vi "2pi_grises.vi"(8 "error in (no error)":errorcluster, 10 "Puerto":refnum<visa-resource-name>="COM2", 11 "Cam Session":T1 caption="Session Out") -> (0 "error out":errorcluster, 3 "V 2Pi\nActual":sgl=3.4309938 format="%#.1g")   [LabVIEW 2020]
uses:
  <vilib>/userdefined/High Color/IMAQdx.ctl
  Controls/Calib states --- typedef.ctl
  Controls/Calib data ---typedef.ctl
  <vilib>/vision/Image Controls.llb/IMAQ Image.ctl
  64c00cdc-7401-4ced-a99b-d285ba44592a.vi
  <vilib>/Instr/_visa.llb/VISA Configure Serial Port (Instr).vi
  <vilib>/vision/driver/NI_Vision_Acquisition_Software.lvlib
  <vilib>/vision/NI_Vision_Development_Module.lvlib
panel:
  out "Last Mouse Position:All Elements":cluster{"X":i32, "Y":i32}
  in  "Sust":bool=TRUE caption="Sustraer?"
  in  "dV (V)":sgl=0.4 min=0.1 max=5 step=0.1 format="%.1f"
  in  "dt (ms)":u32=5
  in  "Rango (V)":u8=7 max=100 step=1
  in  "Canal":string="X"
  in  "Cancelar":bool
  in  "V 2Pi\nApriori":sgl=4.0 min=0.1 max=15 step=0.1 format="%.1f"
  in  "Selección Rectángulo (px)":T2={"Left"=80, "Top"=180, "Right"=730, "Bottom"=830}
  out "valor enviado":string="17.2"
  in  "Iniciar":bool
  out "Captura":T3(plugin-control)
  out "tiempo total":u32=1016
  out "Ciclos 2Pi":cluster{"xi used":dbl[], "yi":dbl[]}[](graph)=[{"xi used"=[0.0, 0.4000000059604645, 0.800000011920929, 1.2000000476837158, 1.600000023841858, 2.0, 2.4000000953674316, 2.799999952316284, 3.200000047683716, 3.6000001430511475, 4.0, 4.400000095367432, 4.800000190734863, 5.200000286102295, 5.599999904632568, 6.0, 6.400000095367432, 6.800000190734863, 7.200000286102295], "yi"=[1.6194082498550415, 2.081223726272583, 3.9639101028442383, 5.417988300323486, 5.994996547698975, 5.763517379760742, 4.927460193634033, 3.268064022064209, 1.9228070974349976, 2.006049633026123, 3.322584629058838, 5.178757190704346, 5.874281883239746, 5.9817633628845215, 5.3586106300354, 3.7743194103240967, 2.4187028408050537, 2.3153183460235596, 3.7917206287384033]}, {"xi used"=[0.0, 0.10000000149011612, 0.20000000298023224, 0.30000000447034836, 0.4000000059604645, 0.5000000074505806, 0.6000000089406967, 0.7000000104308128, 0.800000011920929, 0.9000000208616257, 1.0000000298023224, 1.100000038743019, 1.2000000476837158, 1.3000000417232513, 1.4000000357627869, 1.5000000298023224, 1.600000023841858, 1.7000000178813934, 1.800000011920929, 1.9000000059604645, 2.0, 2.100000023841858, 2.200000047683716, 2.3000000715255737, 2.4000000953674316, 2.5000000596046448, 2.600000023841858, 2.699999988079071, 2.799999952316284, 2.899999976158142, 3.0, 3.100000023841858, 3.200000047683716, 3.3000000715255737, 3.4000000953674316, 3.5000001192092896, 3.6000001430511475, 3.7000001072883606, 3.8000000715255737, 3.900000035762787, 4.0, 4.100000023841858, 4.200000047683716, 4.300000071525574, 4.400000095367432, 4.5000001192092896, 4.6000001430511475, 4.700000166893005, 4.800000190734863, 4.900000214576721, 5.000000238418579, 5.100000262260437, 5.200000286102295, 5.300000190734863, 5.400000095367432, 5.5, 5.599999904632568, 5.699999928474426, 5.799999952316284, 5.899999976158142, 6.0, 6.100000023841858, 6.200000047683716, 6.300000071525574, 6.400000095367432, 6.5000001192092896, 6.6000001430511475, 6.700000166893005, 6.800000190734863, 6.900000214576721, 7.000000238418579, 7.100000262260437, 7.200000286102295], "yi"=[1.6194082498550415, 1.6415202646400873, 1.700969021152869, 1.835091261121122, 2.081223726272583, 2.4615675244221595, 2.9377812277334487, 3.4563877744572187, 3.9639101028442383, 4.416314498578613, 4.807340439884618, 5.1401707620402455, 5.417988300323486, 5.643229129866736, 5.815342479071086, 5.9330308007455095, 5.994996547698975, 6.0015645873541725, 5.959549445588673, 5.8773880628937665, 5.763517379760742, 5.622745854472534, 5.4453682711596425, 5.218050945615625, 4.927460193634033, 4.566549653810085, 4.153420905030226, 3.7124627576598135, 3.268064022064209, 2.8442846434260165, 2.4638706226251452, 2.1492390703865025, 1.9228070974349976, 1.8016579460584699, 1.7815393847964844, 1.8528653137515367, 2.006049633026123, 2.2327082258196134, 2.529265762805696, 2.8933489839101707, 3.322584629058838, 3.807336769827714, 4.308917005977046, 4.78137419407865, 5.178757190704346, 5.467236063197128, 5.661465721984701, 5.788222288265946, 5.874281883239746, 5.940712665430707, 5.985750942666336, 6.001925060099863, 5.9817633628845215, 5.9173299887642, 5.798831744986865, 5.616011126946077, 5.3586106300354, 5.0225638976458455, 4.628571701943094, 4.203526165358669, 3.7743194103240967, 3.3657338746848104, 2.994113257941885, 2.673691575010305, 2.4187028408050537, 2.2430304554985607, 2.1591553602930404, 2.1792078816481535, 2.3153183460235596, 2.5722541809073114, 2.925331217901028, 3.3425023896347215, 3.7917206287384033]}, {"xi used"=[1.6635191881348852, 5.094512955533968], "yi"=[6.004797437208987, 6.001979760925586]}]
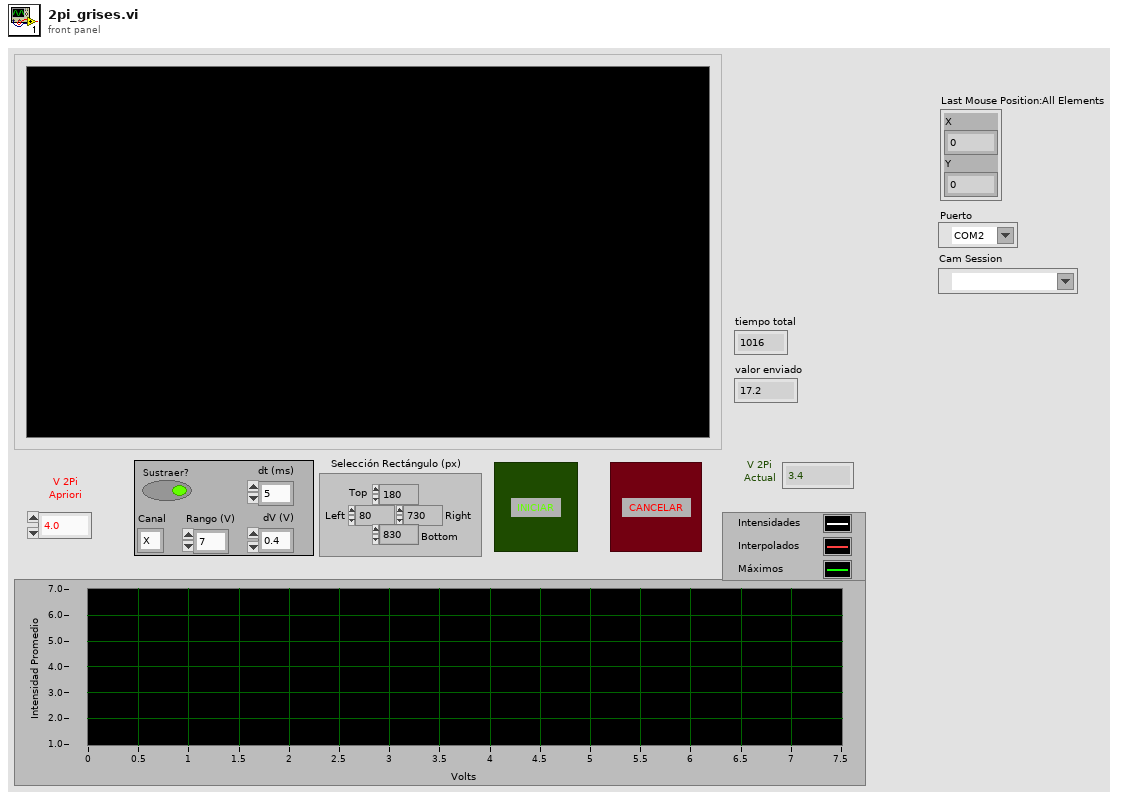
[diagram p1: front panel]
types:
  T1 = typedef "IMAQdx.ctl" = refnum<k21>
  T2 = cluster{"Left":i32, "Top":i32, "Right":i32, "Bottom":i32}
  T3 = typedef "IMAQ Image.ctl" = refnum<image>
  T4 = typedef "Calib data ---typedef.ctl" = cluster{"t0":u32, "Voltage":sgl[], "Mean pix value":sgl[], "Rectangle":cluster{"Left":i32, "Top":i32, "Right":i32, "Bottom":i32}, "New calibration?":bool, "Images":T3[]}
  T5 = typedef "Calib states --- typedef.ctl" = enum16{"Init", "Wait", "Aqcuire base image", "Aquire and process", "Calculate results", "Prompt to repeat", "Clear buffers", "Exit"}
  T6 = typedef "lveventtype.ctl" = enum32{"Null", "Timeout", "Annotation Menu Selection", "Annotation Menu Selection?", "App Instance Close", "App Instance Close?", "Autoscale Range Change", "Bookmark Info Change", "Cell Edit", "Cell Edit?", "Cursor Grab", "Cursor Grab?", "Cursor Menu Selection", "Cursor Menu Selection?", "Cursor Move", "Cursor Release", "Data Change", "Direction Change", "Display State Change", "Drag Ended", "Drag Enter", "Drag Leave", "Drag Over", "Drag Source Update", "Drag Starting", "Drag Starting?", "Drop", "Exec State Change", "Key Down", "Key Down?", "Key Repeat", "Key Repeat?", "Key Up", "Listbox Double Click", "Menu Activation?", "Menu Selection (App)", "Menu Selection? (App)", "Menu Selection (User)", "Mouse Down", "Mouse Down?", "Mouse Enter", "Mouse Leave", "Mouse Move", "Mouse Up", "Mouse Wheel", "NI Security User Change (App)", "Pane Size", "Panel Close", "Panel Close?", "Panel Resize", "Plot Attribute Change", "Scale Range Change", "Shortcut Menu Activation?", "Shortcut Menu Selection (App)", "Shortcut Menu Selection? (App)", "Shortcut Menu Selection (User)", "Tree Double Click", "Tree Drag", "Tree Drag?", "Tree Drop", "Tree Drop?", "Tree Item Close", "Tree Item Close?", "Tree Item Open", "Tree Item Open?", "User Event", "Value Change"}
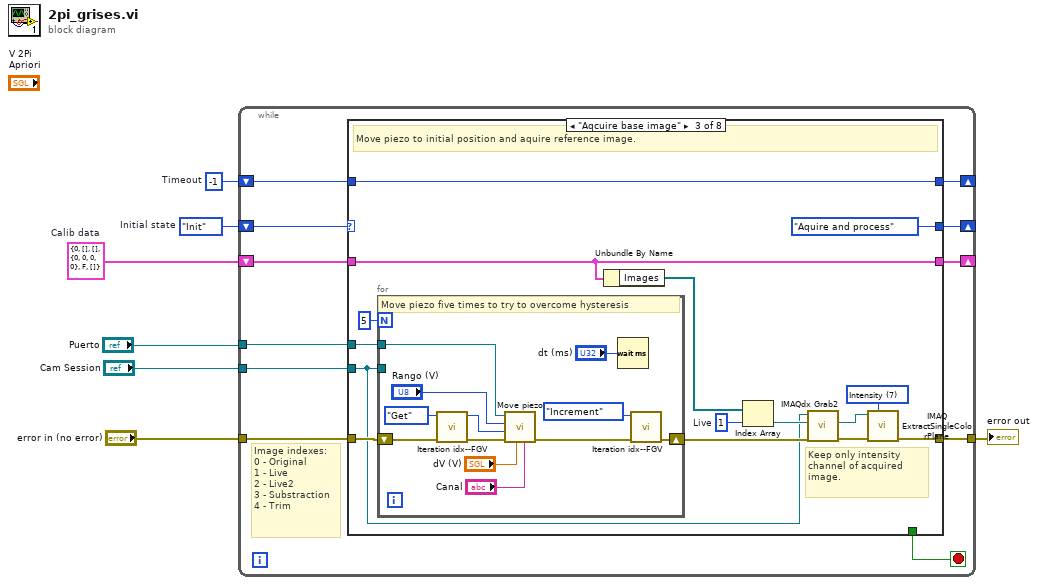
[diagram p0: block diagram]
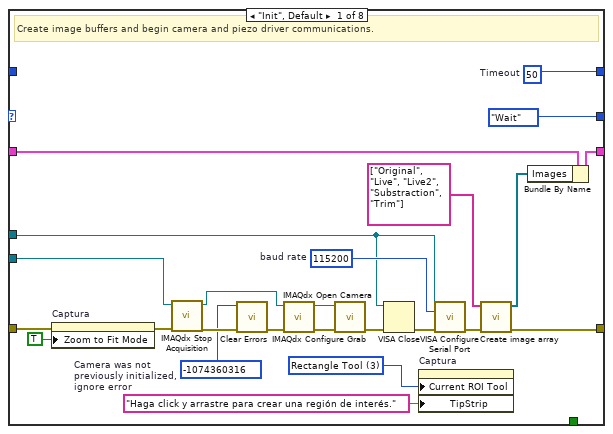
[diagram p2: hidden frame]
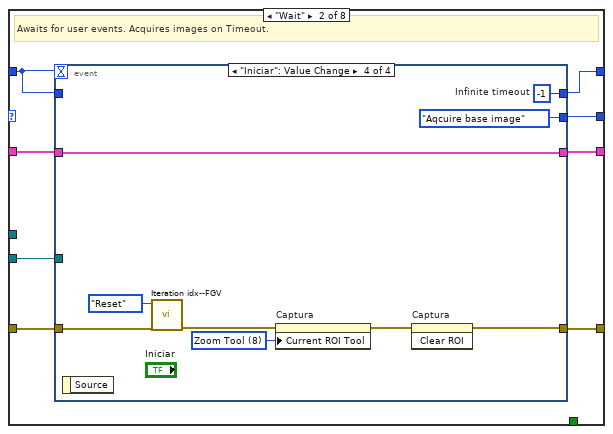
[diagram p3: hidden frame]
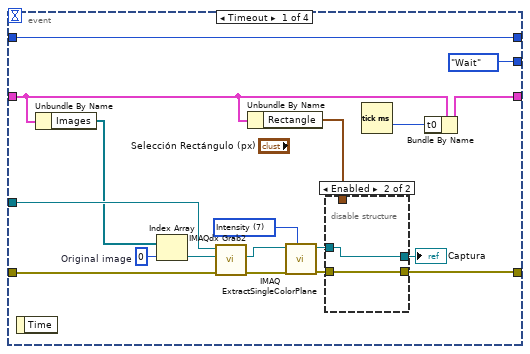
[diagram p4: hidden frame]
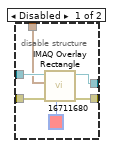
[diagram p5: hidden frame]
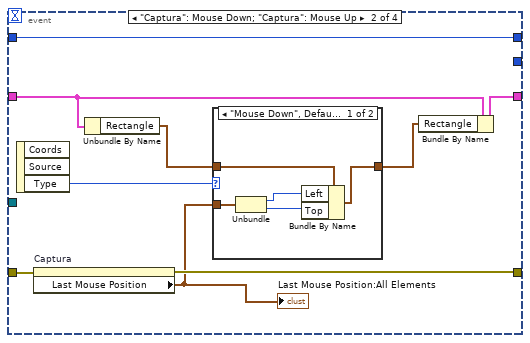
[diagram p6: hidden frame]
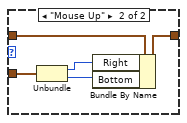
[diagram p7: hidden frame]
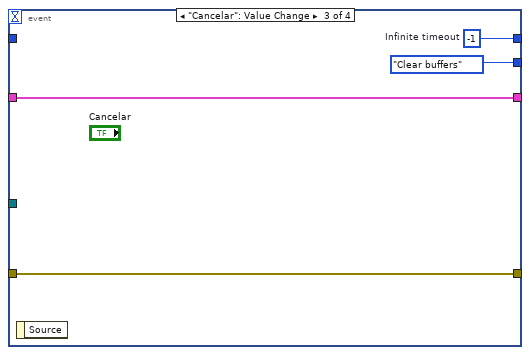
[diagram p8: hidden frame]
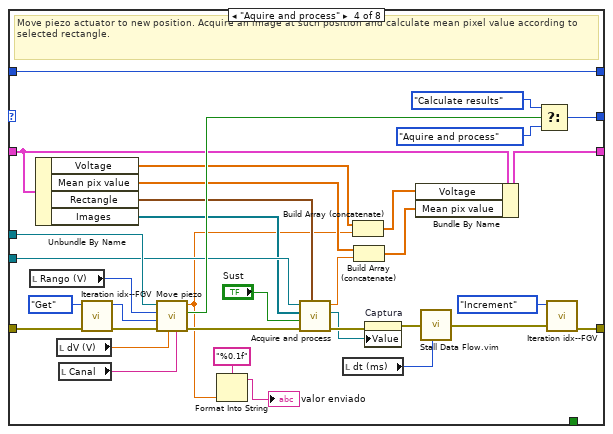
[diagram p9: hidden frame]
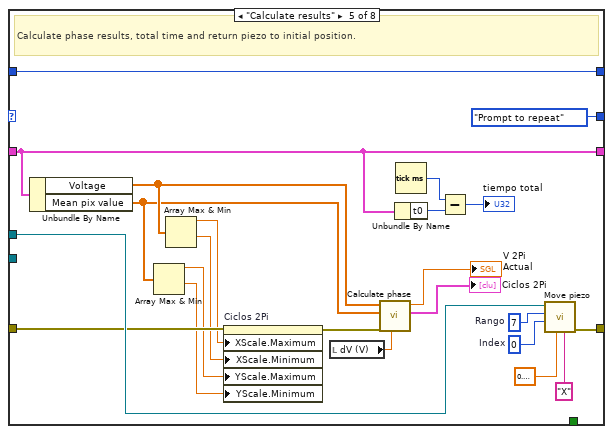
[diagram p10: hidden frame]
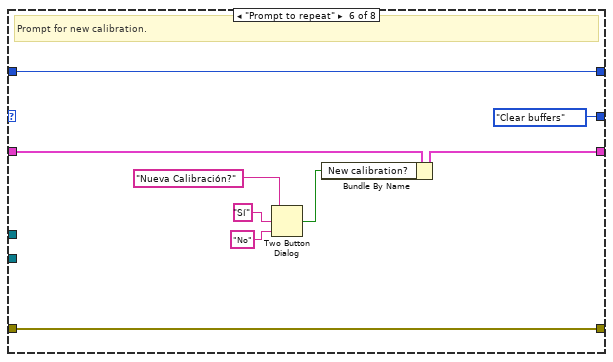
[diagram p11: hidden frame]
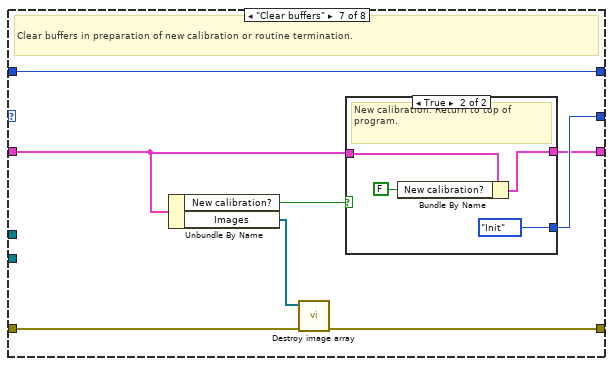
[diagram p12: hidden frame]
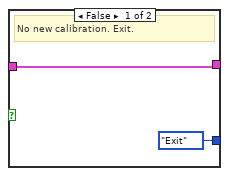
[diagram p13: hidden frame]
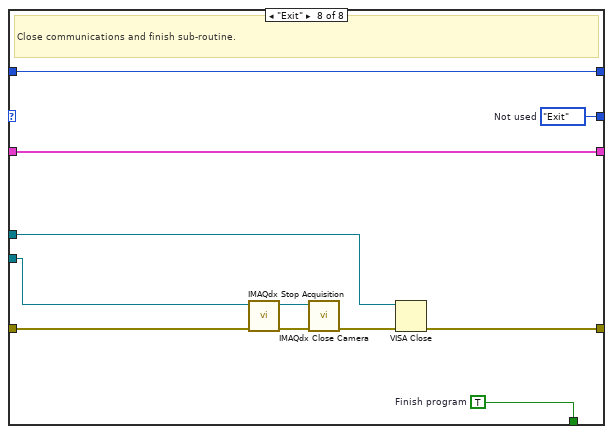
[diagram p14: hidden frame]
diagram:
  w2 = T4 {"t0"=0, "Voltage"=[], "Mean pix value"=[], "Rectangle"={"Left"=0, "Top"=0, "Right"=0, "Bottom"=0}, "New calibration?"=FALSE, "Images"=[]}  # Calib data
  w3 = -1  # Timeout
  w7 = Calib_states_---_typedef."Init"  # Initial state
  n1 = while {
    tunnel: [w16] -> w5
    tunnel: "error in (no error)" -> [w15]
    shift-right: [w14] -> _
    shift-left: w7 -> [w18]
    tunnel: "Cam Session" -> [w13]
    shift-right: [w11] -> _
    shift-left: w3 -> [w12]
    shift-right: [w10] -> _
    shift-left: w2 -> [w9]
    tunnel: "Puerto" -> [w8]
    stop <- w17 stop-if-true
    # "Image indexes:\n0 - Original\n1 - Live\n2 - Live2\n3 - Substraction\n4 - Trim"
    n2 = case shown="\"Aqcuire base image\"" w18 {
      tunnel: [_ _ _ _ _ _ _ w227] -> w17
      tunnel: [w26 w46 w112 w162 w184 w202 w208 w218] -> w16
      tunnel: w15 -> [w32 w47 w122 w168 w178 w202 w209 w223]
      tunnel: [Calib_states_---_typedef."Wait" w50 Calib_states_---_typedef."Aquire and process" ("Not used") w163 Calib_states_---_typedef."Prompt to repeat" ("Not used") Calib_states_---_typedef."Clear buffers" ("f") w210 w226] -> w14
      tunnel: w13 -> [w36 w45 w109 w157 _ _ _ w222]
      tunnel: w12 -> [_ w49 w123 w170 w193 w201 w207 w225]
      tunnel: [w33 w48 w123 w170 w193 w201 w207 w225] -> w11
      tunnel: [w22 w44 w111 w155 w188 w194 w204 w224] -> w10
      tunnel: w9 -> [w23 w43 w111 w154 w188 w196 w205 w224]
      tunnel: w8 -> [w24 _ w119 w169 w183 _ _ w217]
      frame "Init", Default {
        w20 = u32 3 items=["Zoom Tool"=8, "Selection Tool"=0, "Pan Tool"=9, "Point Tool"=1, "Line Tool"=2, "Rectangle Tool"=3, "Rotated Rectangle Tool"=12, "Polyline Tool"=10, "Polygon Tool"=5, "Freehand Tool"=11, "Closed Freehand Tool"=6, "Ellipse Tool"=4, "Annulus Tool"=7] ("Current ROI Tool")
        w30 = u32 115200  # baud rate
        w33 = 50  # Timeout
        w37 = -1074360316  # Camera was not previously initialized, ignore error
        # "Create image buffers and begin camera and piezo driver communications."
        n3 = property on="Captura" class="ImageControl"(error in=w32, "Zoom to Fit Mode"=TRUE) -> (error out=w28:errorcluster)  [unwired: 1 in, 1 out]
        n4 = call <vilib>:"IMAQdx Stop Acquisition.vi"("error in"=w28, "Session In"=w36) -> ("error out"=w40:errorcluster, "Session Out"=w38:T1)  [unwired: 8 in]
        n5 = call <vilib>:"Clear Errors.vi"("error in (no error)"=w40, "specific error code to clear (0: all)"=w37) -> ("error out"=w39:errorcluster)  [unwired: 4 in, 1 out]
        n6 = call <vilib>:"IMAQdx Open Camera.vi"("error in"=w39, "Session In"=w38) -> ("error out"=w35:errorcluster, "Session Out"=w34:T1)  [unwired: 8 in]
        n7 = call <vilib>:"IMAQdx Configure Grab.vi"("error in"=w35, "Session In"=w34) -> ("error out"=w29:errorcluster)  [unwired: 8 in, 1 out]
        n8 = VISA Close(VISA resource name=w24, error in (no error)=w29) -> (error out=w25:errorcluster)
        n9 = property on="Captura" class="ImageControl"("Current ROI Tool"=w20, "TipStrip"="Haga click y arrastre para crear una región de interés." ("Tip Strip")) -> ()  [unwired: 2 in, 2 out]
        n10 = call-poly "VISA Configure Serial Port"("VISA resource name"=w24, "baud rate (9600)"=w30, "error in (no error)"=w25) -> ("error out"=w27:errorcluster)  [unwired: 11 in, 1 out]
        n11 = call "Create image array.vi"("error in (no error)"=w27, "Name idx"=string[] ["Original", "Live", "Live2", "Substraction", "Trim"]) -> ("error out"=w26:errorcluster, "Image array"=w21:T3[])  [unwired: 8 in]
        n12 = Bundle By Name(cluster=w23, "Images"=w21) -> (w22:T4)
      }
      frame "Wait" {
        # "Awaits for user events. Acquires images on Timeout."
        n13 = event shown="[3] \"Iniciar\": Value Change" {
          selector: _ -> [_ _ _ _]
          dyn-events: _ -> [_ _ _ _]
          timeout: w49 -> [_ _ _ _]
          tunnel: [Calib_states_---_typedef."Wait" _ Calib_states_---_typedef."Clear buffers" Calib_states_---_typedef."Aqcuire base image"] -> w50
          tunnel: w49 -> [w67 w85 _ _]
          tunnel: [w67 w85 w96 w106] -> w48
          tunnel: w47 -> [w64 w84 w98 w104]
          tunnel: [w59 w83 w98 w100] -> w46
          tunnel: w45 -> [w63 _ _ _]
          tunnel: [w55 w78 w97 w108] -> w44
          tunnel: w43 -> [w52 w79 w97 w108]
          event Timeout {
            w53 = 7 items=["Red", "Green", "Blue", "Hue", "Saturation", "Luminance", "Value", "Intensity"] ("Color Plane")
            w66 = 0  # Original image
            n14 = event-data() -> ()  [unwired: 1 in, 1 out]
            n15 = Unbundle By Name(w52) -> ("Images"=w54:T3[])
            n16 = Index Array(array=w54, index=w66) -> (element=w65:T3)
            n17 = call <vilib>:"IMAQdx Grab2.vi"("error in"=w64, "Image In"=w65, "Session In"=w63) -> ("error out"=w60:errorcluster, "Image Out"=w57:T3)  [unwired: 5 in, 2 out]
            n18 = Unbundle By Name(w52) -> ("Rectangle"=w51:T2)
            n19 = call "IMAQ ExtractSingleColorPlane"("Color Plane"=w53, "error in (no error)"=w60, "Image Src"=w57) -> ("error out"=w62:errorcluster, "Image Dst Out"=w61:T3)  [unwired: 7 in]
            n20 = disable-structure shown="Enabled" {
              disable-tunnel: w62 -> [w74 w75]
              disable-tunnel: w61 -> [w73 w76]
              disable-tunnel: [w72 w75] -> w59
              disable-tunnel: [w71 w76] -> w58
              disable-tunnel: w51 -> [w69 _]
              frame Disabled {
                n21 = call "IMAQ Overlay Rectangle"("Color"=u32 16711680, "error in (no error)"=w74, "Rectangle"=w69, "Image"=w73) -> ("error out"=w72:errorcluster, "Image Out"=w71:T3)  [unwired: 6 in]
              }
              frame Enabled {
              }
            }
            "Captura" <- w58
            n22 = Tick Count (ms)() -> (millisecond timer value=w56:u32)
            n23 = Bundle By Name(cluster=w52, "t0"=w56) -> (w55:T4)
          }
          event "Captura": Mouse Down; "Captura": Mouse Up {
            n24 = event-data() -> ("Type"=w82:T6)  [unwired: 1 in, 2 out]
            n25 = property on="Captura" class="ImageControl"(error in=w84) -> (error out=w83:errorcluster, "Last Mouse Position"=w80:cluster{"X":i32, "Y":i32})  [unwired: 1 in, 1 out]
            "Last Mouse Position:All Elements" <- w80
            n26 = Unbundle By Name(w79) -> ("Rectangle"=w81:T2)
            n27 = case shown="\"Mouse Down\", Default" w82 {
              tunnel: w81 -> [w87 w94]
              tunnel: w80 -> [w88 w95]
              tunnel: [w86 w91] -> w77
              frame "Mouse Down", Default {
                n28 = Unbundle(w88) -> ("X"=w90:i32, "Y"=w89:i32)
                n29 = Bundle By Name(cluster=w87, "Left"=w90, "Top"=w89) -> (w86:T2)
              }
              frame "Mouse Up" {
                n30 = Unbundle(w95) -> ("X"=w93:i32, "Y"=w92:i32)
                n31 = Bundle By Name(cluster=w94, "Right"=w93, "Bottom"=w92) -> (w91:T2)
              }
            }
            n32 = Bundle By Name(cluster=w79, "Rectangle"=w77) -> (w78:T4)
          }
          event "Cancelar": Value Change {
            w96 = -1  # Infinite timeout
            n33 = event-data() -> ()  [unwired: 1 in, 1 out]
          }
          event "Iniciar": Value Change {
            w102 = u32 8 items=["Zoom Tool"=8, "Selection Tool"=0, "Pan Tool"=9, "Point Tool"=1, "Line Tool"=2, "Rectangle Tool"=3, "Rotated Rectangle Tool"=12, "Polyline Tool"=10, "Polygon Tool"=5, "Freehand Tool"=11, "Closed Freehand Tool"=6, "Ellipse Tool"=4, "Annulus Tool"=7] ("Current ROI Tool")
            w106 = -1  # Infinite timeout
            n34 = event-data() -> ()  [unwired: 1 in, 1 out]
            n35 = call "Iteration idx--FGV.vi"("error in (no error)"=w104, "Action"=enum16{"Reset", "Get", "Increment"}."Reset") -> ("error out"=w103:errorcluster)  [unwired: 8 in, 1 out]
            n36 = property on="Captura" class="ImageControl"(error in=w103, "Current ROI Tool"=w102) -> (error out=w101:errorcluster)  [unwired: 1 in, 1 out]
            n37 = invoke on="Captura" class="ImageControl" method="Clear ROI"(error in=w101) -> (error out=w100:errorcluster)  [unwired: 2 in, 2 out]
          }
        }
      }
      frame "Aqcuire base image" {
        w116 = 7 items=["Red", "Green", "Blue", "Hue", "Saturation", "Luminance", "Value", "Intensity"] ("Color Plane")
        w115 = 1  # Live
        # "Keep only intensity channel of acquired image."
        # "Move piezo to initial position and aquire reference image."
        n38 = for {
          N: 5 -> [_]
          tunnel: w109 -> [_]
          shift-right: [w133] -> w114
          shift-left: w122 -> [w132]
          tunnel: w119 -> [w128]
          # "Move piezo five times to try to overcome hysteresis"
          n39 = call "Iteration idx--FGV.vi"("error in (no error)"=w132, "Action"=enum16{"Reset", "Get", "Increment"}."Get") -> ("error out"=w130:errorcluster, "Index"=w124:i32)  [unwired: 8 in]
          n40 = call "Move piezo.vi"("Canal"="Canal", "dV"="dV (V)", "error in (no error)"=w130, "Index"=w124, "Rango"="Rango (V)", "VISA Refnum in"=w128) -> ("error out"=w129:errorcluster)  [unwired: 3 in, 2 out]
          n41 = Wait (ms)(milliseconds to wait="dt (ms)") -> ()  [unwired: 1 out]
          n42 = call "Iteration idx--FGV.vi"("error in (no error)"=w129, "Action"=enum16{"Reset", "Get", "Increment"}."Increment") -> ("error out"=w133:errorcluster)  [unwired: 8 in, 1 out]
        }
        n43 = Unbundle By Name(w111) -> ("Images"=w110:T3[])
        n44 = Index Array(array=w110, index=w115) -> (element=w118:T3)
        n45 = call <vilib>:"IMAQdx Grab2.vi"("error in"=w114, "Image In"=w118, "Session In"=w109) -> ("error out"=w113:errorcluster, "Image Out"=w117:T3)  [unwired: 5 in, 2 out]
        n46 = call "IMAQ ExtractSingleColorPlane"("Color Plane"=w116, "error in (no error)"=w113, "Image Src"=w117) -> ("error out"=w112:errorcluster)  [unwired: 7 in, 1 out]
      }
      frame "Aquire and process" {
        # "Move piezo actuator to new position. Acquire an image at such position and calculate mean pixel value according to selected rectangle."
        n47 = local read "Rango (V)"() -> (w138:u8)
        n48 = Unbundle By Name(w154) -> ("Voltage"=w153:sgl[], "Mean pix value"=w150:sgl[], "Rectangle"=w151:T2, "Images"=w144:T3[])
        n49 = local read "dV (V)"() -> (w137:sgl)
        n50 = local read "Canal"() -> (w136:string)
        n51 = call "Iteration idx--FGV.vi"("error in (no error)"=w168, "Action"=enum16{"Reset", "Get", "Increment"}."Get") -> ("error out"=w167:errorcluster, "Index"=w159:i32)  [unwired: 8 in]
        n52 = call "Move piezo.vi"("Canal"=w136, "dV"=w137, "error in (no error)"=w167, "Index"=w159, "Rango"=w138, "VISA Refnum in"=w169) -> ("error out"=w158:errorcluster, "Stop?"=w160:bool, "Voltage"=w139:sgl)  [unwired: 3 in]
        n53 = Format Into String(format string="%0.1f", w139) -> (resulting string=→"valor enviado":string)  [unwired: 2 in, 1 out]
        n54 = call "Acquire and process.vi"("Rectangle"=w151, "error in (no error)"=w158, "Substract images?"="Sust", "Image array"=w144, "Cam session"=w157) -> ("error out"=w147:errorcluster, "Trimmed image"=w145:T3, "Mean Value"=w149:sgl)  [unwired: 4 in]
        n55 = local read "dt (ms)"() -> (w142:u32)
        n56 = Build Array (concatenate)(w153, w139) -> (w152:sgl[])
        n57 = Build Array (concatenate)(w150, w149) -> (w148:sgl[])
        n58 = property on="Captura" class="ImageControl"(error in=w147, "Value"=w145) -> (error out=w146:errorcluster)  [unwired: 1 in, 1 out]
        n59 = Bundle By Name(cluster=w154, "Voltage"=w152, "Mean pix value"=w148) -> (w155:T4)
        n60 = call "Stall Data Flow.vim"("value in"=w146, "milliseconds to wait"=w142) -> ("value out"=w143:errorcluster)  [unwired: 1 out]
        n61 = Select(t=Calib_states_---_typedef."Calculate results" ("Not used"), s=w160, f=Calib_states_---_typedef."Aquire and process") -> (s? t:f=w163:T5)
        n62 = call "Iteration idx--FGV.vi"("error in (no error)"=w143, "Action"=enum16{"Reset", "Get", "Increment"}."Increment") -> ("error out"=w162:errorcluster)  [unwired: 8 in, 1 out]
      }
      frame "Calculate results" {
        w179 = u8 7  # Rango
        w180 = 0  # Index
        # "Calculate phase results, total time and return piezo to initial position."
        n63 = Unbundle By Name(w188) -> ("Voltage"=w176:sgl[], "Mean pix value"=w173:sgl[])
        n64 = Array Max & Min(array=w173) -> (max value=w172:sgl, min value=w171:sgl)  [unwired: 2 out]
        n65 = Array Max & Min(array=w176) -> (max value=w175:sgl, min value=w174:sgl)  [unwired: 2 out]
        n66 = property on="Ciclos 2Pi" class="XYGraph (strict)"(error in=w178, "XScale.Maximum"=w175, "XScale.Minimum"=w174, "YScale.Maximum"=w172, "YScale.Minimum"=w171) -> (error out=w177:errorcluster)  [unwired: 1 in, 1 out]
        n67 = local read "dV (V)"() -> (w190:sgl)
        n68 = call "Calculate phase.vi"("dV (V)"=w190, "error in (no error)"=w177, "Mean values"=w173, "Voltages"=w176) -> ("Ciclos 2Pi 2"=→"Ciclos 2Pi":cluster{"xi used":dbl[], "yi":dbl[]}[], "V 2Pi\nActual 2"=→"V 2Pi\nActual":sgl)  [unwired: 5 in, 1 out]
        n69 = Unbundle By Name(w188) -> ("t0"=w186:u32)
        n70 = Tick Count (ms)() -> (millisecond timer value=w187:u32)
        n71 = Subtract(x=w187, y=w186) -> (x-y=→"tiempo total":u32)
        n72 = call "Move piezo.vi"("Canal"="X", "dV"=sgl 0.4, "Index"=w180, "Rango"=w179, "VISA Refnum in"=w183) -> ("error out"=w184:errorcluster)  [unwired: 4 in, 2 out]
      }
      frame "Prompt to repeat" {
        # "Prompt for new calibration."
        n73 = Two Button Dialog(message="Nueva Calibración?", 1:"No" ("F button name (\"Cancel\")"), 2:"Sí" ("F button name (\"Cancel\")")) -> (T button?=w195:bool)
        n74 = Bundle By Name(cluster=w196, "New calibration?"=w195) -> (w194:T4)
      }
      frame "Clear buffers" {
        # "Clear buffers in preparation of new calibration or routine termination."
        n75 = Unbundle By Name(w205) -> ("New calibration?"=w206:bool, "Images"=w203:T3[])
        n76 = call "Destroy image array.vi"("error in (no error)"=w209, "Image array"=w203) -> ("error out"=w208:errorcluster)  [unwired: 9 in]
        n77 = case shown="True" w206 {
          tunnel: [Calib_states_---_typedef."Exit" Calib_states_---_typedef."Init"] -> w210
          tunnel: w205 -> [w212 w215]
          tunnel: [w212 w213] -> w204
          frame False {
            # "No new calibration. Exit."
          }
          frame True {
            # "New calibration. Return to top of program."
            n78 = Bundle By Name(cluster=w215, "New calibration?"=FALSE) -> (w213:T4)
          }
        }
      }
      frame "Exit" {
        w226 = Calib_states_---_typedef."Exit"  # Not used
        w227 = TRUE  # Finish program
        # "Close communications and finish sub-routine."
        n79 = call <vilib>:"IMAQdx Stop Acquisition.vi"("error in"=w223, "Session In"=w222) -> ("error out"=w221:errorcluster, "Session Out"=w220:T1)  [unwired: 8 in]
        n80 = call <vilib>:"IMAQdx Close Camera.vi"("error in"=w221, "Session In"=w220) -> ("error out"=w219:errorcluster)  [unwired: 9 in]
        n81 = VISA Close(VISA resource name=w217, error in (no error)=w219) -> (error out=w218:errorcluster)
      }
    }
  }
  "error out" <- w5
